vi "LargeRandomNumber (SubVI).vi"() -> (3 "Random Number":string)   [LabVIEW 2011]
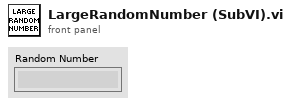
[diagram p1: front panel]
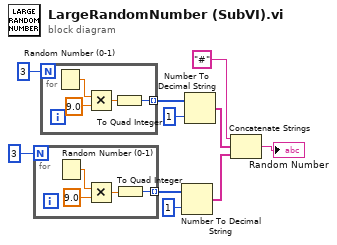
[diagram p0: block diagram]
diagram:
  n1 = for {
    N: 3 ("Numeric") -> [_]
    tunnel: [w11] -> w7 mode=indexing
    n2 = Random Number (0-1)() -> (number: 0 to 1=w13:dbl)
    n3 = Multiply(x=w13, y=9.0) -> (x*y=w12:dbl)
    n4 = To Quad Integer(1:w12) -> (0:w11:i64)
  }
  n5 = for {
    N: 3 ("Numeric") -> [_]
    tunnel: [w15] -> w4 mode=indexing
    n6 = Random Number (0-1)() -> (number: 0 to 1=w17:dbl)
    n7 = Multiply(x=w17, y=9.0) -> (x*y=w16:dbl)
    n8 = To Quad Integer(1:w16) -> (0:w15:i64)
  }
  n9 = Number To Decimal String(number=w7, width (-)=i16 1) -> (decimal integer string=w8:string[])
  n10 = Number To Decimal String(number=w4, width (-)=i16 1) -> (decimal integer string=w9:string[])
  n11 = Concatenate Strings("#", w9, w8) -> (→"Random Number":string)
